vi "Simple Quit Verification.vi"() -> ()   [LabVIEW 2020, in "Dialog Boxes.lvlib"]
uses:
  Dialog Boxes.lvlib
  toolbox/Standard Signalling/ude_Stop Application/Get Event Reference.vi
  toolbox/Standard Signalling/ude_Stop Application/ude_Stop Application.lvlib
panel:
  in  "No":bool
  in  "Yes":bool
  # "You are about to shutdown the application. Are you sure this is what you want to do?"
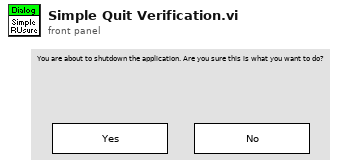
[diagram p1: front panel]
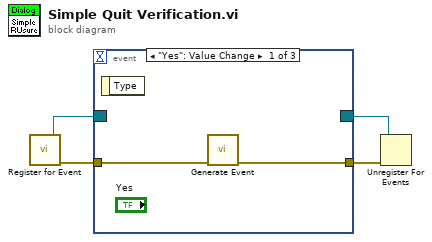
[diagram p0: block diagram]
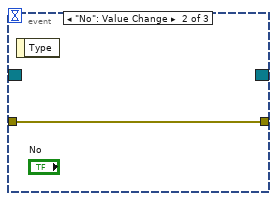
[diagram p2: hidden frame]
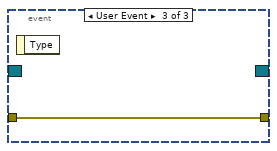
[diagram p3: hidden frame]
diagram:
  n1 = call "Register for Event.vi"() -> ("Error Out"=w3:errorcluster, "sys"=w4:refnum<event-registration>)  [unwired: 6 in]
  n2 = event shown="[0] \"Yes\": Value Change" {
    selector: w4 -> [_ _ _]
    dyn-events: [_ _ _] -> w1
    timeout: _ -> [_ _ _]
    tunnel: w3 -> [w6 w7 w8]
    tunnel: [w5 w7 w8] -> w2
    event "Yes": Value Change {
      n3 = event-data() -> ()  [unwired: 1 in, 1 out]
      n4 = call "Generate Event.vi"("Error In"=w6) -> ("Error Out"=w5:errorcluster)  [unwired: 6 in]
    }
    event "No": Value Change {
      n5 = event-data() -> ()  [unwired: 1 in, 1 out]
    }
    event User Event {
      n6 = event-data() -> ()  [unwired: 1 in, 1 out]
    }
  }
  n7 = Unregister For Events(event registration refnum=w1, error in=w2) -> ()  [unwired: 1 out]
